vi "Error_ObtainErrorQueue.vi"(1 "Enum":enum16{"Init", "ReturnQueueRef"}(ring)=enum."ReturnQueueRef", 5 "error in (no error)":errorcluster) -> (14 "ErrorQueue":refnum<queue>, 19 "error out":errorcluster)   [LabVIEW 2017]
doc: "Obtains a queue of size 10 containing error clusters on the first call. Thereafter returns this queue."
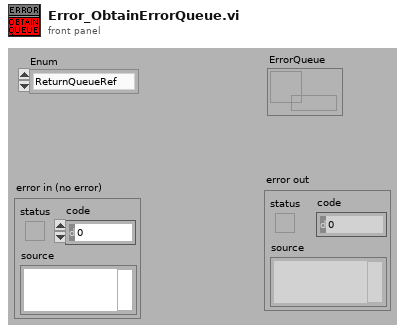
[diagram p1: front panel]
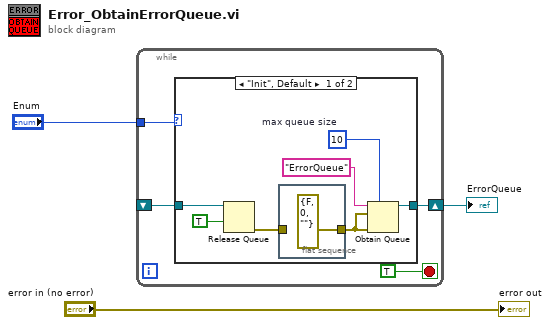
[diagram p0: block diagram]
diagram:
  n1 = while {
    shift-right: [w7] -> w2
    shift-left: _ -> [w6]
    tunnel: "Enum" -> [w4]
    stop <- TRUE stop-if-true
    n2 = case shown="\"Init\", Default" w4 {
      tunnel: [w12 w16] -> w7
      tunnel: w6 -> [w11 w16]
      frame "Init", Default {
        w14 = 10  # max queue size
        n3 = Release Queue(queue=w11, force destroy? (F)=TRUE) -> (error out=w9:errorcluster)  [unwired: 1 in, 2 out]
        n4 = flat-sequence {
          tunnel: [errorcluster {"status"=FALSE, "code"=0, "source"=""} ("error in (no error)")] -> w8
          tunnel: w9 -> [_]
          frame #0 {
          }
        }
        n5 = Obtain Queue(max queue size (-1, unlimited)=w14, name (unnamed)="ErrorQueue", element data type=w8, error in (no error)=w8) -> (queue out=w12:refnum<queue>)  [unwired: 1 in, 2 out]
      }
      frame "ReturnQueueRef" {
      }
    }
  }
  "ErrorQueue" <- w2
  "error out" <- "error in (no error)"
